vi "Field_and_Temperature_sweep_at the same _time.vi"   [LabVIEW 2019]
uses:
  Monitors/Utility/Monitor Communication/LS370/LS370-Control.ctl
  Global/Global Variables/global.vi
  Instrument_Setup.vi
  Monitors/Utility/Monitor Communication/sub-vis/16T_Open_Queue.vi
  Global/Global Variables/Data_Display_global.vi
  Monitors/Utility/Monitor Communication/sub-vis/16T_Queue_Commands.vi
  Monitors/Utility/Monitor Communication/sub-vis/20T_Open_Queue.vi
  Monitors/Utility/Monitor Communication/sub-vis/20T_Queue_Commands.vi
  Monitors/Utility/Monitor Communication/sub-vis/LS370_Open_Queue.vi
  Monitors/Utility/Monitor Communication/sub-vis/VTI_Open_Queue.vi
  Monitors/Utility/Monitor Communication/sub-vis/VTI_Queue_Commands.vi
types:
  T1 = typedef "LS370-Control.ctl" = cluster{"Disable Heater":bool, "Activate Tsweep":bool, "Update Lakeshores":bool, "Setpoint - Manual":dbl, "Rate (K/min)":dbl, "Sorb Power (mW)":dbl, "Still Power (mW)":dbl, "Sorb Heater":bool, "Still Heater":bool, "Set Temperature Sweep Main":bool}
  T2 = typedef "16T-Cluster.ctl" = cluster{"Clamp":bool, "Switch Heater":bool, "Go to Zero":bool, "Go to set":bool, "Go to Hold":bool, "Clamped":bool, "Quenched":bool, "Rate limit":bool, "Persistent":bool, "Hold":bool, "Set":bool, "Zero":bool, "Magnet (T)":dbl, "Leads (T)":dbl, "Magnet T (K)":dbl, "Switch":bool, "Setpoint (T)":dbl, "Rate (T/min)":dbl, "Select":bool, "Sweeping":bool}
  T3 = typedef "16T_Control.ctl" = cluster{"Clamp":bool, "Switch Heater":bool, "Go to Zero":bool, "Go to Set":bool, "Go to Hold":bool, "Setpoint (T)":dbl, "Rate (T/min)":dbl, "Set Rate":bool}
  T4 = typedef "15T-Cluster.ctl" = cluster{"Magnet (T)":dbl, "Leads (T)":dbl, "Setpoint (T)":dbl, "Rate (T/min)":dbl, "Set":bool, "Zero":bool, "Hold":bool, "Go to zero":bool, "Go to Hold":bool, "Go to Set":bool, "Clamp":bool, "Switch Heater":bool, "Rate limit":bool, "Switch":bool, "Clamped":bool, "Persistent":bool, "Quenched":bool, "Sweeping":bool, "Select":bool}
  T5 = typedef "15T-Control.ctl" = cluster{"Setpoint (T)":dbl, "Rate (T/min)":dbl, "Go to zero":bool, "Go to Hold":bool, "Go to Set":bool, "Clamp":bool, "Switch Heater":bool}
  T6 = typedef "20T_Cluster.ctl" = cluster{"Clamp":bool, "Switch Heater":bool, "Go to Zero":bool, "Go to set":bool, "Go to Hold":bool, "Clamped":bool, "Hold":bool, "Set":bool, "Zero":bool, "Magnet (T)":dbl, "Leads (T)":dbl, "Magnet T (K)":dbl, "Switch":bool, "Target Field (T)":dbl, "Field Setpoint (T)":dbl, "Rate Setpoint (T/min)":dbl, "Set Rate":bool, "Rate\n(T/min) ":dbl, "lambda NV (%)":dbl, "lambda p (mbar)":dbl, "lambda-Control":bool, "Activate lambda control":bool, "lambda NV  SP":dbl, "Set lambda NV":bool, "PSU Status":string, "PSU\nVoltage":dbl}
  T7 = typedef "20T_Control.ctl" = cluster{"Clamp":bool, "Switch Heater":bool, "Go to Zero":bool, "Go to Set":bool, "Go to Hold":bool, "Field Setpoint (T)":dbl, "Rate Setpoint (T/min)":dbl, "Set Rate":bool, "Activate lambda control":bool, "Set lambda NV":bool, "lambda NV  SP":dbl}
  T8 = typedef "5T-Cluster.ctl" = cluster{"Go to set":bool, "Go to Zero":bool, "Clamp":bool, "Go to Hold":bool, "Clamped ":bool, "Quenched 2":bool, "Rate limit 2":bool, "Magnet (T)":dbl, "Leads (T)":dbl, "Rate (T/min)":dbl, "Sweeping":bool, "Setpoint":dbl, "Set":bool, "Zero":bool, "Hold":bool, "Clamp":bool}
  T9 = typedef "5T_Control.ctl" = cluster{"Rate (T/min)":dbl, "Setpoint":dbl, "Go to set":bool, "Go to Zero":bool, "Clamp":bool, "Go to Hold":bool, "Set Rate":bool}
  T10 = typedef "LS372-Cluster.ctl" = cluster{"Activate Tsweep":bool, "Setpoint - Manual":dbl, "Rate (K/min)":dbl, "Update Lakeshores":bool, "Still Heater":bool, "Still Power (mW)":dbl, "Manual Heater":bool, "Manual Heater  (mW) ":dbl, "Heater Range":dbl, "P (Gain)":dbl, "I (Reset)":dbl, "D (Rate)":dbl, "Heater Power (mW)":dbl, "MC Thermometer":u16, "MC Temperature":dbl, "LS372-T1":dbl, "LS372 -T2":dbl, "LS372-R1 ":dbl, "LS372-R2":dbl, "LS372-T3":dbl, "LS372-T4":dbl, "LS372-R3 ":dbl, "LS372-R4 \n\n\n\n":dbl, "LS372-T5":dbl, "LS372-T6":dbl, "LS372-R5":dbl, "LS372-R6 ":dbl, "Still Power ist":dbl, "Set Temperatur Sweep main":bool, "Setpoint ist":dbl, "Disable Heater":bool}
  T11 = typedef "Ls372-Control.ctl" = cluster{"Activate Tsweep":bool, "Setpoint - Manual":dbl, "Rate (K/min)":dbl, "Update Lakeshores":bool, "Still Heater":bool, "Still Power (mW)":dbl, "Manual Heater":bool, "Manual Heater  (mW) ":dbl, "MC Thermometer":u16, "Set Temperature Sweeep main":bool, "Disable Heater":bool}
  T12 = typedef "VTI-cluster.ctl" = cluster{"Temperatur (K)":dbl, "Setpoint (K)":dbl, "Rate (K/min)":dbl, "Heater (%)":dbl, "NV (%)":dbl, "Heater Manual":bool, "NV Manual":bool, "Go to Set":bool, "Pressure":dbl, "Heater SP":dbl, "Valid?":bool, "Set Heater SP":bool, "Set NV SP":bool, "Heater (%) Display":dbl, "NV (%) Display":dbl, "NV Setpoint":dbl, "Change Heater Status":bool, "Change NV Status":bool, "Sample 3":dbl, "Sample 2":dbl, "Sweep-State":bool, "Set Auto PID":bool, "Auto PID":bool, "Stopp":bool, "Setpoint-Sweep":dbl}
  T13 = typedef "VTI-control.ctl" = cluster{"Set VTI SP":bool, "Change NV Status":bool, "Set NV Setpoint":bool, "Change Heater Status":bool, "Set Heater Setpoint":bool, "Setpoint (K)":dbl, "Rate (K/min)":dbl, "Setpoint Heater":dbl, "Setpoint NV":dbl, "Change Auto PID":bool, "Stop Sweep":bool}
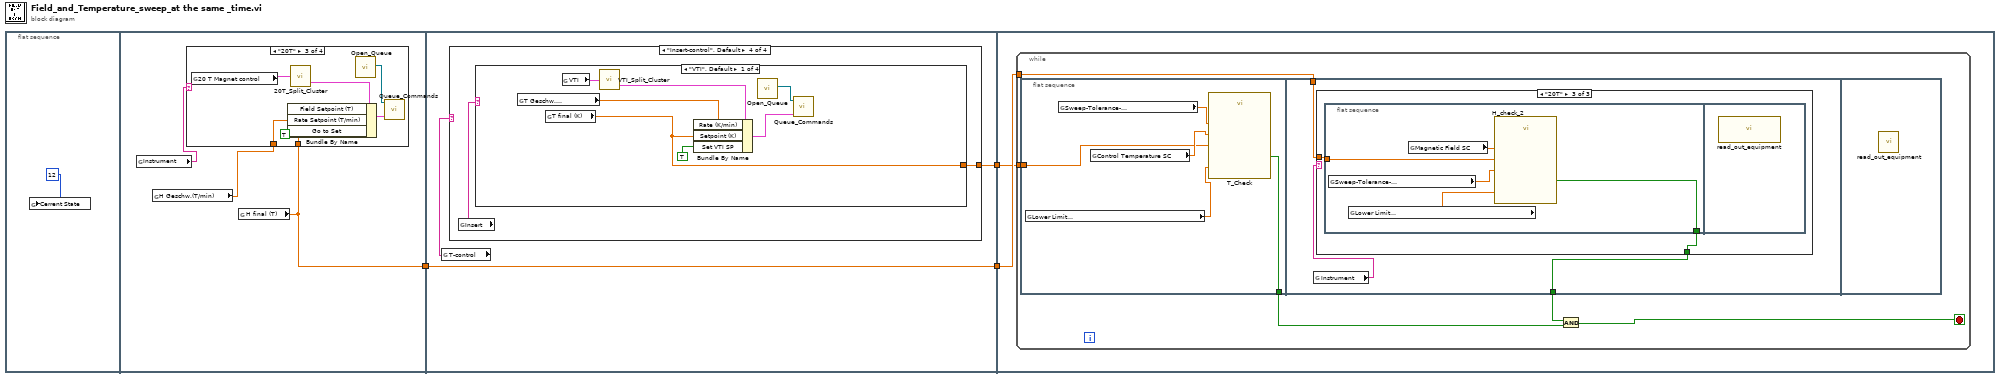
[diagram p0: block diagram]
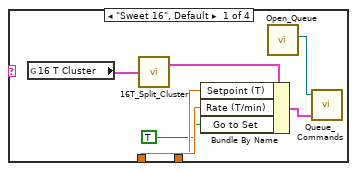
[diagram p2: hidden frame]
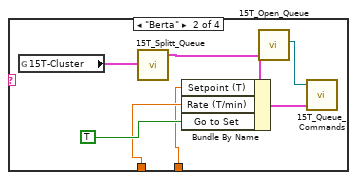
[diagram p3: hidden frame]
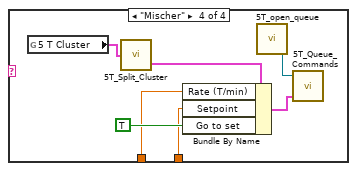
[diagram p4: hidden frame]
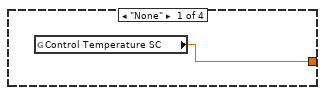
[diagram p5: hidden frame]
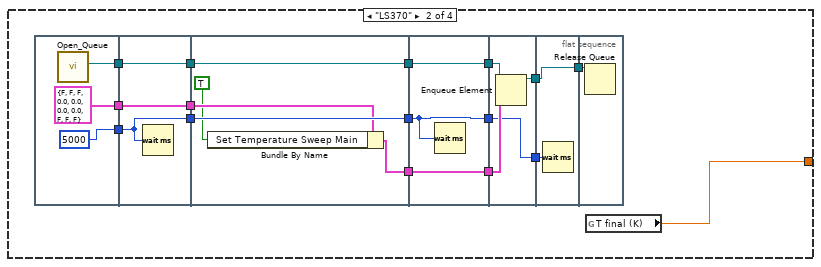
[diagram p6: hidden frame]
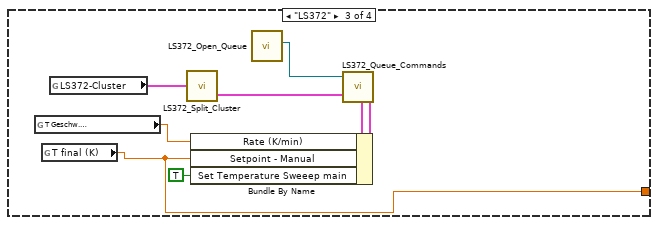
[diagram p7: hidden frame]
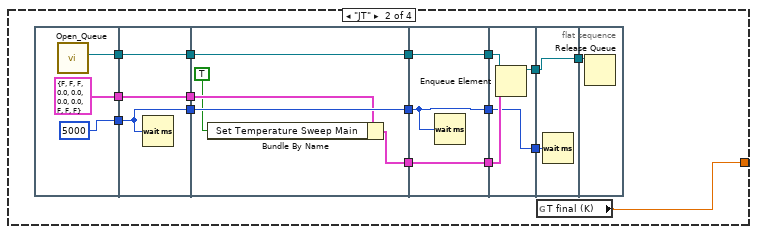
[diagram p8: hidden frame]
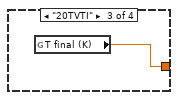
[diagram p9: hidden frame]
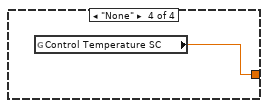
[diagram p10: hidden frame]
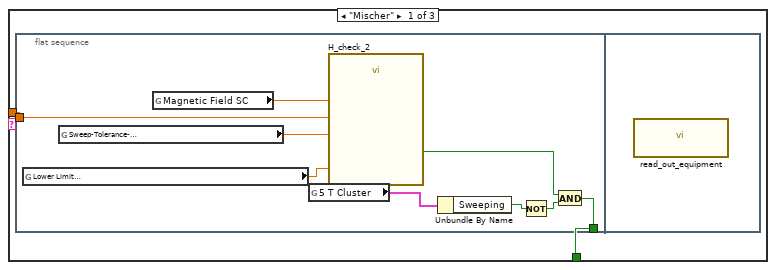
[diagram p11: hidden frame]
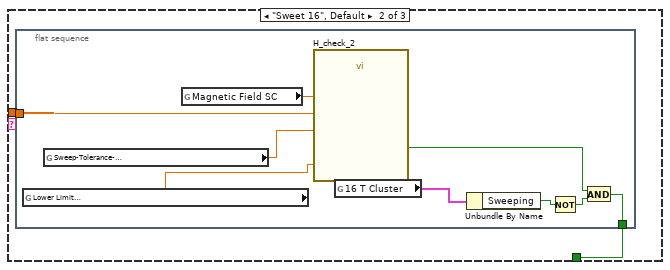
[diagram p12: hidden frame]
diagram:
  n1 = flat-sequence {
    tunnel: [w5] -> w2
    tunnel: [w37] -> w3
    tunnel: w2 -> [w37]
    tunnel: [w36] -> w1
    tunnel: w3 -> [w133]
    tunnel: w1 -> [w132]
    frame #0 {
      n2 = global write "global.vi" "Cerrent State"(12) -> ()
    }
    frame #1 {
      n3 = global read "Instrument_Setup.vi" "Instrument"() -> (w6:string)
      n4 = global read "global.vi" "H Geschw.(T/min)"() -> (w7:dbl)
      n5 = global read "global.vi" "H final (T)"() -> (w5:dbl)
      n6 = case shown="\"20T\"" w6 {
        tunnel: w7 -> [w12 w16 w24 w30]
        tunnel: w5 -> [w11 w15 w23 w29]
        frame "Sweet 16", Default {
          n7 = global read "Data_Display_global.vi" "16 T Cluster"() -> (w13:T2)
          n8 = call "16T_Split_Cluster.vi"("16 T Magnet control"=w13) -> ("16 T Magnet control"=w10:T3)  [unwired: 1 out]
          n9 = Bundle By Name(cluster=w10, "Setpoint (T)"=w11, "Rate (T/min)"=w12, "Go to Set"=TRUE) -> (w9:T3)
          n10 = call-poly "Open_Queue.vi"() -> ("queue out"=w14:refnum<queue>)  [unwired: 10 in, 1 out]
          n11 = call-poly "Queue_Commands.vi"("16 T Magnet control"=w9, "16T Queue"=w14) -> ()  [unwired: 1 in, 1 out]
        }
        frame "Berta" {
          n12 = global read "Data_Display_global.vi" "15T-Cluster"() -> (w20:T4)
          n13 = call "15T_Splitt_Queue.vi"("15T-Cluster"=w20) -> ("15T-Control"=w19:T5)  [unwired: 1 in, 1 out]
          n14 = Bundle By Name(cluster=w19, "Setpoint (T)"=w15, "Rate (T/min)"=w16, "Go to Set"=TRUE) -> (w17:T5)
          n15 = call "15T_Open_Queue.vi"() -> ("queue out"=w21:refnum<queue>)  [unwired: 10 in, 1 out]
          n16 = call "15T_Queue_Commands.vi"("15T-Control"=w17, "15T Queue"=w21) -> ()  [unwired: 1 in, 1 out]
        }
        frame "20T" {
          n17 = global read "Data_Display_global.vi" "20 T Magnet control"() -> (w27:T6)
          n18 = call "20T_Split_Cluster.vi"("20 T Cluster"=w27) -> ("20 T Control"=w25:T7)  [unwired: 1 out]
          n19 = Bundle By Name(cluster=w25, "Field Setpoint (T)"=w23, "Rate Setpoint (T/min)"=w24, "Go to Set"=TRUE) -> (w26:T7)
          n20 = call-poly "Open_Queue.vi"() -> ("queue out"=w28:refnum<queue>)  [unwired: 10 in, 1 out]
          n21 = call-poly "Queue_Commands.vi"("20T Control (in)"=w26, "20T Queue"=w28) -> ()  [unwired: 1 in, 1 out]
        }
        frame "Mischer" {
          n22 = global read "Data_Display_global.vi" "5 T Cluster"() -> (w35:T8)
          n23 = call "5T_Split_Cluster.vi"("5 T Cluster"=w35) -> ("5T Control"=w34:T9)  [unwired: 1 out]
          n24 = Bundle By Name(cluster=w34, "Rate (T/min)"=w30, "Setpoint"=w29, "Go to set"=TRUE) -> (w33:T9)
          n25 = call "5T_open_queue.vi"() -> ("queue out"=w32:refnum<queue>)  [unwired: 10 in, 1 out]
          n26 = call "5T_Queue_Commands.vi"("5T Control"=w33, "5T Queue"=w32) -> ()  [unwired: 1 in, 1 out]
        }
      }
    }
    frame #2 {
      n27 = global read "Instrument_Setup.vi" "T-control"() -> (w38:string)
      n28 = case shown="\"Insert-control\", Default" w38 {
        tunnel: [w39 w40 w77 w84] -> w36
        frame "None" {
          n29 = global read "Data_Display_global.vi" "Control Temperature SC"() -> (w39:dbl)
        }
        frame "LS370" {
          n30 = flat-sequence {
            tunnel: [w58] -> w55
            tunnel: [5000] -> w54
            tunnel: [T1 {"Disable Heater"=FALSE, "Activate Tsweep"=FALSE, "Update Lakeshores"=FALSE, "Setpoint - Manual"=0.0, "Rate (K/min)"=0.0, "Sorb Power (mW)"=0.0, "Still Power (mW)"=0.0, "Sorb Heater"=FALSE, "Still Heater"=FALSE, "Set Temperature Sweep Main"=FALSE} ("JT-Cluster")] -> w53
            tunnel: w55 -> [w61]
            tunnel: w54 -> [w60]
            tunnel: [w61] -> w52
            tunnel: [w60] -> w51
            tunnel: [w59] -> w50
            tunnel: w53 -> [w59]
            tunnel: w52 -> [w66]
            tunnel: w51 -> [w65]
            tunnel: w50 -> [w64]
            tunnel: [w66] -> w49
            tunnel: [w65] -> w48
            tunnel: [w62] -> w47
            tunnel: w49 -> [w69]
            tunnel: w48 -> [w68]
            tunnel: w47 -> [w67]
            tunnel: [w69] -> w46
            tunnel: [w68] -> w45
            tunnel: [w67] -> w44
            tunnel: w46 -> [w73]
            tunnel: w45 -> [w70]
            tunnel: w44 -> [w72]
            tunnel: [w71] -> w43
            tunnel: [w70] -> w42
            tunnel: w43 -> [w75]
            tunnel: [w75] -> w41
            tunnel: w42 -> [w74]
            tunnel: w41 -> [w76]
            frame #0 {
              n31 = call-poly "Open_Queue.vi"() -> ("queue out"=w58:refnum<queue>)  [unwired: 10 in, 1 out]
            }
            frame #1 {
              n32 = Wait (ms)(milliseconds to wait=w60) -> ()  [unwired: 1 out]
            }
            frame #2 {
              n33 = Bundle By Name(cluster=w64, "Set Temperature Sweep Main"=TRUE) -> (w62:T1)
            }
            frame #3 {
              n34 = Wait (ms)(milliseconds to wait=w68) -> ()  [unwired: 1 out]
            }
            frame #4 {
              n35 = Enqueue Element(queue=w73, element=w72) -> (queue out=w71:refnum<queue>)  [unwired: 2 in, 2 out]
            }
            frame #5 {
              n36 = Wait (ms)(milliseconds to wait=w74) -> ()  [unwired: 1 out]
            }
            frame #6 {
              n37 = Release Queue(queue=w76) -> ()  [unwired: 2 in, 3 out]
            }
          }
          n38 = global read "global.vi" "T final (K)"() -> (w40:dbl)
        }
        frame "LS372" {
          n39 = global read "global.vi" "T Geschw. \n(K/min)"() -> (w80:dbl)
          n40 = global read "global.vi" "T final (K)"() -> (w77:dbl)
          n41 = global read "Data_Display_global.vi" "LS372-Cluster"() -> (w83:T10)
          n42 = call "LS372_Split_Cluster.vi"("LS372-Cluster"=w83) -> ("LS372-Control"=w82:T11)  [unwired: 1 out]
          n43 = Bundle By Name(cluster=w82, "Rate (K/min)"=w80, "Setpoint - Manual"=w77, "Set Temperature Sweeep main"=TRUE) -> (w78:T11)
          n44 = call "LS372_Open_Queue.vi"() -> ("queue out"=w79:refnum<queue>)  [unwired: 10 in, 1 out]
          n45 = call "LS372_Queue_Commands.vi"("LS372-Control"=w78, "Queue"=w79) -> ()  [unwired: 1 in, 1 out]
        }
        frame "Insert-control", Default {
          n46 = global read "Instrument_Setup.vi" "Insert"() -> (w85:string)
          n47 = case shown="\"VTI\", Default" w85 {
            tunnel: [w86 w93 w130 w131] -> w84
            frame "VTI", Default {
              n48 = global read "global.vi" "T Geschw. \n(K/min)"() -> (w87:dbl)
              n49 = global read "global.vi" "T final (K)"() -> (w86:dbl)
              n50 = global read "Data_Display_global.vi" "VTI"() -> (w91:T12)
              n51 = call "VTI_Split_Cluster.vi"("VTI"=w91) -> ("VTI Control"=w90:T13)  [unwired: 1 out]
              n52 = Bundle By Name(cluster=w90, "Rate (K/min)"=w87, "Setpoint (K)"=w86, "Set VTI SP"=TRUE) -> (w89:T13)
              n53 = call-poly "Open_Queue.vi"() -> ("queue out"=w92:refnum<queue>)  [unwired: 10 in, 1 out]
              n54 = call-poly "Queue_Commands.vi"("VTI Control"=w89, "20TVTI Queue"=w92) -> ()  [unwired: 1 in, 1 out]
            }
            frame "JT" {
              n55 = flat-sequence {
                tunnel: [w111] -> w108
                tunnel: [5000] -> w107
                tunnel: [T1 {"Disable Heater"=FALSE, "Activate Tsweep"=FALSE, "Update Lakeshores"=FALSE, "Setpoint - Manual"=0.0, "Rate (K/min)"=0.0, "Sorb Power (mW)"=0.0, "Still Power (mW)"=0.0, "Sorb Heater"=FALSE, "Still Heater"=FALSE, "Set Temperature Sweep Main"=FALSE} ("JT-Cluster")] -> w103
                tunnel: w108 -> [w114]
                tunnel: w107 -> [w113]
                tunnel: [w114] -> w106
                tunnel: [w113] -> w105
                tunnel: [w112] -> w104
                tunnel: w103 -> [w112]
                tunnel: w106 -> [w119]
                tunnel: w105 -> [w118]
                tunnel: w104 -> [w117]
                tunnel: [w119] -> w102
                tunnel: [w118] -> w101
                tunnel: [w115] -> w100
                tunnel: w102 -> [w122]
                tunnel: w101 -> [w121]
                tunnel: w100 -> [w120]
                tunnel: [w122] -> w99
                tunnel: [w121] -> w98
                tunnel: [w120] -> w97
                tunnel: w99 -> [w126]
                tunnel: w98 -> [w123]
                tunnel: w97 -> [w125]
                tunnel: [w124] -> w96
                tunnel: [w123] -> w94
                tunnel: w96 -> [w128]
                tunnel: [w128] -> w95
                tunnel: w94 -> [w127]
                tunnel: w95 -> [w129]
                frame #0 {
                  n56 = call-poly "Open_Queue.vi"() -> ("queue out"=w111:refnum<queue>)  [unwired: 10 in, 1 out]
                }
                frame #1 {
                  n57 = Wait (ms)(milliseconds to wait=w113) -> ()  [unwired: 1 out]
                }
                frame #2 {
                  n58 = Bundle By Name(cluster=w117, "Set Temperature Sweep Main"=TRUE) -> (w115:T1)
                }
                frame #3 {
                  n59 = Wait (ms)(milliseconds to wait=w121) -> ()  [unwired: 1 out]
                }
                frame #4 {
                  n60 = Enqueue Element(queue=w126, element=w125) -> (queue out=w124:refnum<queue>)  [unwired: 2 in, 2 out]
                }
                frame #5 {
                  n61 = Wait (ms)(milliseconds to wait=w127) -> ()  [unwired: 1 out]
                }
                frame #6 {
                  n62 = Release Queue(queue=w129) -> ()  [unwired: 2 in, 3 out]
                }
              }
              n63 = global read "global.vi" "T final (K)"() -> (w93:dbl)
            }
            frame "20TVTI" {
              n64 = global read "global.vi" "T final (K)"() -> (w130:dbl)
            }
            frame "None" {
              n65 = global read "Data_Display_global.vi" "Control Temperature SC"() -> (w131:dbl)
            }
          }
        }
      }
    }
    frame #3 {
      n66 = while {
        tunnel: w133 -> [w135]
        tunnel: w132 -> [w134]
        stop <- w138 stop-if-true
        n67 = flat-sequence {
          tunnel: [w142] -> w137
          tunnel: w134 -> [w140]
          tunnel: [w145] -> w136
          tunnel: w135 -> [w144]
          frame #0 {
            n68 = global read "Instrument_Setup.vi" "Lower Limit\nSweep-Tolerance-\nTemperature (K)"() -> (w139:dbl)
            n69 = global read "Instrument_Setup.vi" "Sweep-Tolerance-\nTemperature (%)"() -> (w143:dbl)
            n70 = global read "Data_Display_global.vi" "Control Temperature SC"() -> (w141:dbl)
            n71 = call "T_Check.vi"("Lower Limit Sweep\nTolerance (K)"=w139, "T_target (K)"=w140, "Sweep\nTolerance %"=w143, "T_in"=w141) -> ("= T target"=w142:bool)
          }
          frame #1 {
            n72 = global read "Instrument_Setup.vi" "Instrument"() -> (w146:string)
            n73 = case shown="\"20T\"" w146 {
              tunnel: [w147 w159 w169] -> w145
              tunnel: w144 -> [w148 w158 w170]
              frame "Mischer" {
                n74 = flat-sequence {
                  tunnel: [w152] -> w147
                  tunnel: w148 -> [w155]
                  frame #0 {
                    n75 = global read "Instrument_Setup.vi" "Lower Limit\nSweep-Tolerance-\nMagnetic-Field (T)"() -> (w149:dbl)
                    n76 = global read "Instrument_Setup.vi" "Sweep-Tolerance-\nMagnetic-Field (%)"() -> (w157:dbl)
                    n77 = global read "Data_Display_global.vi" "Magnetic Field SC"() -> (w156:dbl)
                    n78 = global read "Data_Display_global.vi" "5 T Cluster"() -> (w154:T8)
                    n79 = call "H_check_2.vi"("Lower Limit\nSweep\nTolerance (T)"=w149, "Sweep\nTolerance %"=w157, "H_in"=w156, "H_target (K)"=w155) -> ("= H target"=w153:bool)  [unwired: 7 in]
                    n80 = Unbundle By Name(w154) -> ("Sweeping"=w150:bool)
                    n81 = Not(x=w150) -> (.not. x?=w151:bool)
                    n82 = And(x=w153, y=w151) -> (x .and. y?=w152:bool)
                  }
                  frame #1 {
                    n83 = call "read_out_equipment.vi"() -> ()  [unwired: 1 in]
                  }
                }
              }
              frame "Sweet 16", Default {
                n84 = flat-sequence {
                  tunnel: [w164] -> w159
                  tunnel: w158 -> [w167]
                  frame #0 {
                    n85 = global read "Instrument_Setup.vi" "Lower Limit\nSweep-Tolerance-\nMagnetic-Field (T)"() -> (w160:dbl)
                    n86 = global read "Instrument_Setup.vi" "Sweep-Tolerance-\nMagnetic-Field (%)"() -> (w161:dbl)
                    n87 = global read "Data_Display_global.vi" "Magnetic Field SC"() -> (w168:dbl)
                    n88 = call "H_check_2.vi"("Lower Limit\nSweep\nTolerance (T)"=w160, "Sweep\nTolerance %"=w161, "H_in"=w168, "H_target (K)"=w167) -> ("= H target"=w165:bool)  [unwired: 7 in]
                    n89 = global read "Data_Display_global.vi" "16 T Cluster"() -> (w166:T2)
                    n90 = Unbundle By Name(w166) -> ("Sweeping"=w162:bool)
                    n91 = Not(x=w162) -> (.not. x?=w163:bool)
                    n92 = And(x=w165, y=w163) -> (x .and. y?=w164:bool)
                  }
                }
              }
              frame "20T" {
                n93 = flat-sequence {
                  tunnel: [w173] -> w169
                  tunnel: w170 -> [w174]
                  frame #0 {
                    n94 = global read "Instrument_Setup.vi" "Sweep-Tolerance-\nMagnetic-Field (%)"() -> (w171:dbl)
                    n95 = global read "Instrument_Setup.vi" "Lower Limit\nSweep-Tolerance-\nMagnetic-Field (T)"() -> (w172:dbl)
                    n96 = global read "Data_Display_global.vi" "Magnetic Field SC"() -> (w175:dbl)
                    n97 = call "H_check_2.vi"("Lower Limit\nSweep\nTolerance (T)"=w172, "Sweep\nTolerance %"=w171, "H_in"=w175, "H_target (K)"=w174) -> ("= H target"=w173:bool)  [unwired: 7 in]
                  }
                  frame #1 {
                    n98 = call "read_out_equipment.vi"() -> ()  [unwired: 1 in]
                  }
                }
              }
            }
          }
          frame #2 {
            n99 = call "read_out_equipment.vi"() -> ()  [unwired: 1 in]
          }
        }
        n100 = And(x=w136, y=w137) -> (x .and. y?=w138:bool)
      }
    }
  }
